vi "GetInterfaceParents.vi"(8 "error in (no error)":errorcluster, 10 "KeepRefsOpen":bool, 11 "LVClassLibrary in":refnum<vi>) -> (0 "error out":errorcluster, 1 "InterfaceParents(Path)":path[](array[path]), 2 "InterfaceParents(Refs)":refnum<vi>[](array[refnum]), 3 "LVClassLibrary Out":refnum<vi>)   [LabVIEW 2020, in "InterfaceLibrary.lvlib"]
uses:
  <resource>/Framework/Providers/Open_GDS/ClassProviders/Common/InterfaceLibrary/InterfaceLibrary.lvlib
  356edce9-d305-4b2d-9913-c89f155d0a74.vi
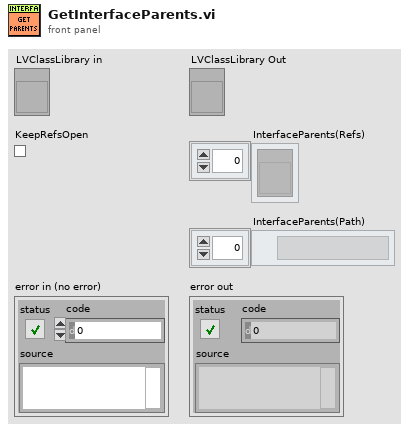
[diagram p1: front panel]
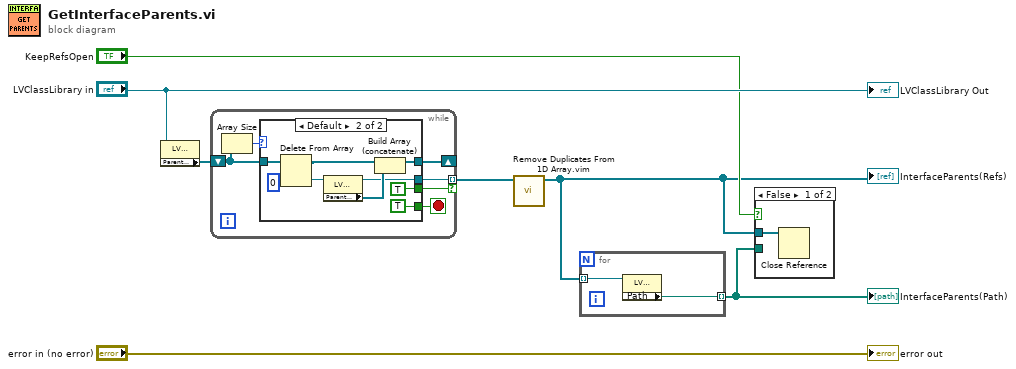
[diagram p0: block diagram]
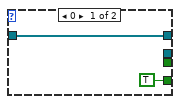
[diagram p3: hidden frame]
diagram:
  n1 = property class="LVClassLibrary"(reference="LVClassLibrary in") -> ("Parent Interfaces"=w7:refnum<vi>[])  [unwired: 1 in, 2 out]
  n2 = while {
    shift-right: [w11] -> _
    shift-left: w7 -> [w13]
    tunnel: [w10] -> w5 mode=indexing if=w9
    stop <- w8 stop-if-true
    n3 = Array Size(array=w13) -> (size(s)=w12:i32)
    n4 = case shown="Default" w12 {
      tunnel: w13 -> [w15 w23]
      tunnel: [w15 w20] -> w11
      tunnel: [_ w18] -> w10
      tunnel: [_ TRUE] -> w9
      tunnel: [TRUE TRUE] -> w8
      frame 0 {
      }
      frame Default {
        n5 = Delete From Array(array=w23, index=0) -> (deleted portion=w21:refnum<vi>, array with subset deleted=w22:refnum<vi>[])  [unwired: 1 in]
        n6 = property class="LVClassLibrary"(reference=w21) -> (reference out=w18:refnum<vi>, "Parent Interfaces"=w19:refnum<vi>[])  [unwired: 1 in, 1 out]
        n7 = Build Array (concatenate)(w22, w19) -> (w20:refnum<vi>[])
      }
    }
  }
  n8 = call "Remove Duplicates From 1D Array.vim"("array"=w5) -> ("array with duplicates removed"=w2:refnum<vi>[])  [unwired: 10 in]
  "InterfaceParents(Refs)" <- w2
  n9 = for {
    tunnel: w2 -> [w26] mode=indexing
    tunnel: [w25] -> w1 mode=indexing
    n10 = property class="LVClassLibrary"(reference=w26) -> ("Path"=w25:path)  [unwired: 1 in, 2 out]
  }
  "InterfaceParents(Path)" <- w1
  n11 = case shown="False" "KeepRefsOpen" {
    tunnel: w2 -> [w27 _]
    tunnel: w1 -> [_ _]
    frame False {
      n12 = Close Reference(reference=w27) -> ()  [unwired: 1 in, 1 out]
    }
    frame True {
    }
  }
  "error out" <- "error in (no error)"
  "LVClassLibrary Out" <- "LVClassLibrary in"
